vi "Temperature Simulator.vi"(11 "error in (no error)":errorcluster) -> (4 "data":dbl, 15 "error out":errorcluster)   [LabVIEW 2015]
doc: "This VI generated a temperature reading and a voltage reading on a sine wave at 50kHz for 5000 points. This VI is used as a simulation in the Weather Station project when no hardware is available."
uses:
  Instance           1 29Saved   Temperature Simulator .vi
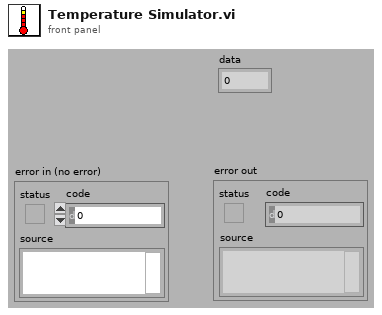
[diagram p1: front panel]
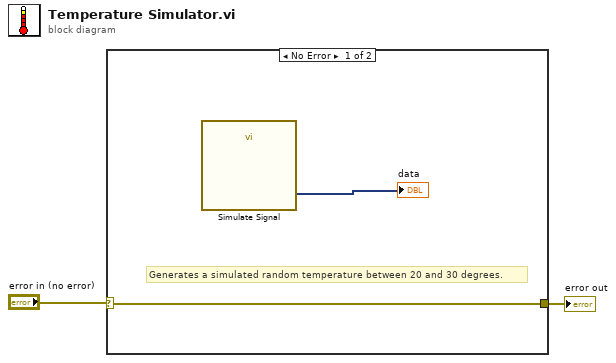
[diagram p0: block diagram]
diagram:
  n1 = case shown="No Error" "error in (no error)" {
    selector: "error in (no error)" -> [w4 w5]
    tunnel: [w4 w5] -> w1
    frame No Error {
      # "Generates a simulated random temperature between 20 and 30 degrees."
      n2 = call "Simulate Signal"() -> ("Temperature"=→"data":dynamicdata)  [unwired: 14 in, 1 out]
    }
    frame Error {
    }
  }
  "error out" <- w1
